vi "23384_Davis_Poku_Amankwa_Amankwa.DavisPoku.MNE1201.2.5_348253_1081795104.vi"() -> ()   [LabVIEW 2018]
panel:
  in  "Blinks Per Minute":dbl
  in  "stop":bool
  out "LED":bool
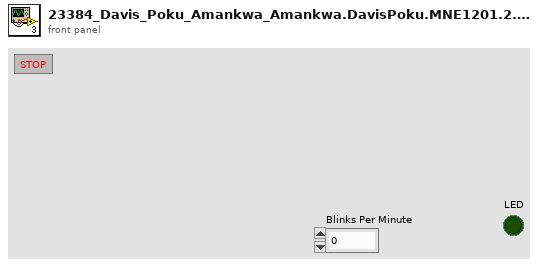
[diagram p1: front panel]
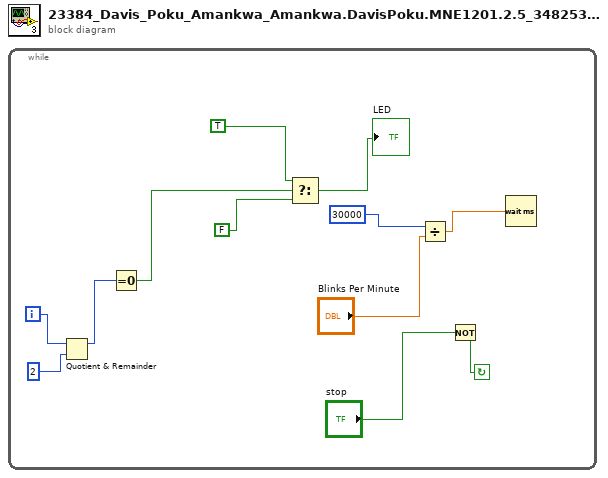
[diagram p0: block diagram]
diagram:
  n1 = while {
    i -> [w7]
    stop <- w11 continue-if-true
    n2 = Quotient & Remainder(x=w7, y=2) -> (x-y*floor(x/y)=w5:i32)  [unwired: 1 out]
    n3 = Equal To 0?(x=w5) -> (x = 0?=w4:bool)
    n4 = Select(t=TRUE, s=w4, f=FALSE) -> (s? t:f=→"LED":bool)
    n5 = Divide(x=30000, y="Blinks Per Minute") -> (x/y=w3:dbl)
    n6 = Not(x="stop") -> (.not. x?=w11:bool)
    n7 = Wait (ms)(milliseconds to wait=w3) -> ()  [unwired: 1 out]
  }
